vi "Create Quoted Filepath.vi"(10 "Path":path) -> (2 "Quoted Path String":string)   [LabVIEW 2014, in "NIPM_API.lvlib"]
doc: "Creates valid command line filepath string for the given Path"
uses:
  NIPM_API.lvlib
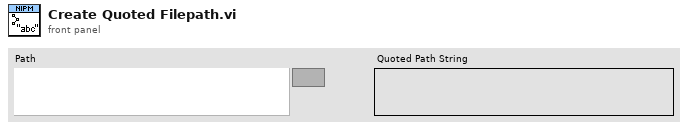
[diagram p1: front panel]
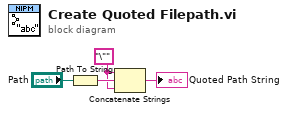
[diagram p0: block diagram]
diagram:
  w2 = "\"" ("string")
  n1 = Path To String(path="Path") -> (string=w4:string)
  n2 = Concatenate Strings(w2, w4, w2) -> (→"Quoted Path String":string)
